vi "LimpaErro.vi"(8 "error in (no error)":errorcluster, 11 "Numeric":i32) -> (0 "error out":errorcluster)   [LabVIEW 2012]
doc: "Esse VI limpa um erro específico. Ele faz a limpeza apenas do erro que possui o código que lhe foi enviado como argumento."
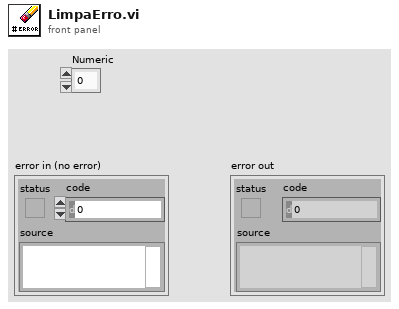
[diagram p1: front panel]
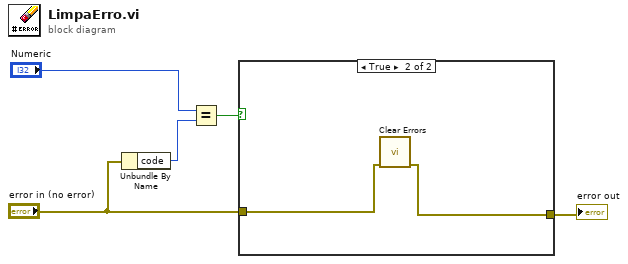
[diagram p0: block diagram]
diagram:
  n1 = Unbundle By Name("error in (no error)") -> ("code"=w5:i32)
  n2 = Equal?(x="Numeric", y=w5) -> (x = y?=w2:bool)
  n3 = case shown="True" w2 {
    tunnel: "error in (no error)" -> [w6 w8]
    tunnel: [w6 w7] -> w1
    frame False {
    }
    frame True {
      n4 = call <vilib>:"Clear Errors.vi"("error in (no error)"=w8) -> ("error out"=w7:errorcluster)  [unwired: 6 in]
    }
  }
  "error out" <- w1
